vi "Voice Init.vi"(8 "Error In":errorcluster, 10 "CMD List":string[](array[string]), 11 "Main Control Reference":T2) -> (0 "Error Out":errorcluster, 3 "Callback Event Reference":T1)   [LabVIEW 2018]
uses:
  Data Def/Voice Control Reference.ctl
  Data Def/Callback Event Reference.ctl
  System.Speech
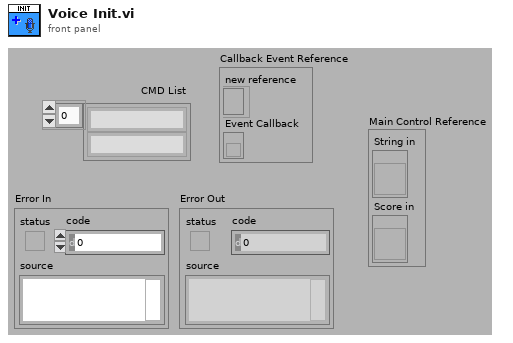
[diagram p1: front panel]
types:
  T1 = typedef "Callback Event Reference.ctl" = cluster{"new reference":refnum<k24>, "Event Callback":refnum<k27>}
  T2 = typedef "Voice Control Reference.ctl" = cluster{"String in":refnum<vi>, "Score in":refnum<vi>}
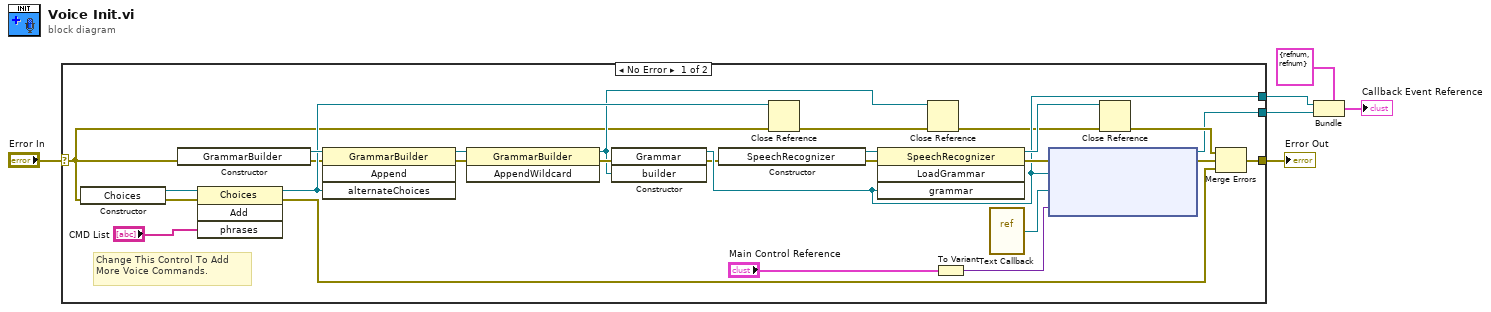
[diagram p0: block diagram]
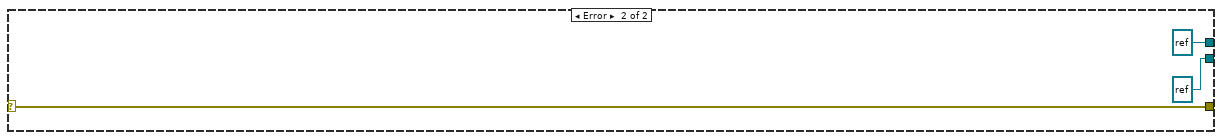
[diagram p2: hidden frame]
diagram:
  n1 = case shown="No Error" "Error In" {
    selector: "Error In" -> [w18 w36]
    tunnel: [w11 refnum<k27> refnum ("Event Callback")] -> w4
    tunnel: [w21 refnum<k24> refnum ("new reference")] -> w3
    tunnel: [w16 w36] -> w5
    frame No Error {
      # "Change This Control To Add More Voice Commands."
      n2 = constructor class="Choices"(error in=w18) -> (reference out=w27:refnum<k24>, error out=w29:errorcluster)  [unwired: 2 in, 1 out]
      n3 = constructor class="GrammarBuilder"(error in=w18) -> (reference out=w25:refnum<k24>, error out=w13:errorcluster)  [unwired: 2 in, 1 out]
      n4 = invoke class="Choices" method="Add"(reference=w27, error in=w29, "phrases"="CMD List") -> (reference out=w24:refnum<k24>, error out=w12:errorcluster)  [unwired: 1 in, 2 out]
      n5 = invoke class="GrammarBuilder" method="Append"(reference=w25, error in=w13, "alternateChoices"=w24) -> (reference out=w28:refnum<k24>, error out=w26:errorcluster)  [unwired: 1 in, 2 out]
      n6 = invoke class="GrammarBuilder" method="AppendWildcard"(reference=w28, error in=w26) -> (reference out=w23:refnum<k24>, error out=w30:errorcluster)  [unwired: 1 in, 1 out]
      n7 = constructor class="Grammar"(error in=w30, "builder"=w23) -> (reference out=w21:refnum<k24>, error out=w10:errorcluster)  [unwired: 2 in, 2 out]
      n8 = constructor class="SpeechRecognizer"(error in=w10) -> (reference out=w32:refnum<k24>, error out=w33:errorcluster)  [unwired: 2 in, 1 out]
      n9 = Close Reference(reference=w24, error in (no error)=w18) -> (error out=w19:errorcluster)
      n10 = invoke class="SpeechRecognizer" method="LoadGrammar"(reference=w32, error in=w33, "grammar"=w21) -> (reference out=w22:refnum<k24>, error out=w31:errorcluster)  [unwired: 1 in, 2 out]
      n11 = Close Reference(reference=w23, error in (no error)=w19) -> (error out=w20:errorcluster)
      n12 = To Variant(anything="Main Control Reference") -> (Variant=w7:variant)
      n13 = vi-ref "Text Callback.vi"() -> (w9:refnum<vi>)
      n14 = node(w31, w21, w9, w7) -> (w11:refnum<k27>, w15:errorcluster)  [unwired: 1 in]
      n15 = Close Reference(reference=w22, error in (no error)=w20) -> (error out=w17:errorcluster)
      n16 = Merge Errors(w17, w15, w12) -> (w16:errorcluster)
    }
    frame Error {
    }
  }
  "Error Out" <- w5
  n17 = Bundle(cluster=T1 {"new reference"=refnum, "Event Callback"=refnum}, "new reference"=w3, "Event Callback"=w4) -> (→"Callback Event Reference":T1)
